vi "Global Variables.vi"() -> ()   [LabVIEW 2012]
panel:
  in  "Pivots Enabled?":bool=TRUE
  in  "Climbing":bool
  in  "Caterpillar Back":bool
  in  "Caterpillar ON":bool
  in  "J2 Xbox RB":bool
  in  "J2 Xbox B":bool
  in  "J2 Xbox Y":bool
  in  "J1 Xbox B":bool
  in  "J2 Xbox X":bool
  in  "J1 Xbox Y":bool
  in  "Climb Shoot Motor":dbl
  in  "J1 Xbox X":bool
  in  "J2 Xbox LB":bool
  in  "J2 Xbox A":bool
  in  "J2 Xbox Select":bool
  in  "J1 Xbox Select":bool
  in  "J1 Xbox LB":bool
  in  "J1 Xbox RB":bool
  in  "J1 Xbox A":bool
  in  "ICE BR":dbl
  in  "ICE BL":dbl
  in  "ICE FR":dbl
  in  "ICE FL":dbl
  in  "Konami":bool
  in  "Calibration BR":dbl
  in  "Calibration BL":dbl
  in  "Calibration FR":dbl
  in  "Calibration FL":dbl
  in  "Rotational Motor BR":dbl
  in  "Rotational Motor BL":dbl
  in  "Rotational Motor FR":dbl
  in  "Rotational Motor FL":dbl
  in  "Drive Motor BR":dbl
  in  "Drive Motor BL":dbl
  in  "Drive Motor FR":dbl
  in  "Drive Motor FL":dbl
  # "Steering"
  # "Drive"
  # "Calibration"
  # "ICE Calibrate"
  # "Buttons"
  # "ICE"
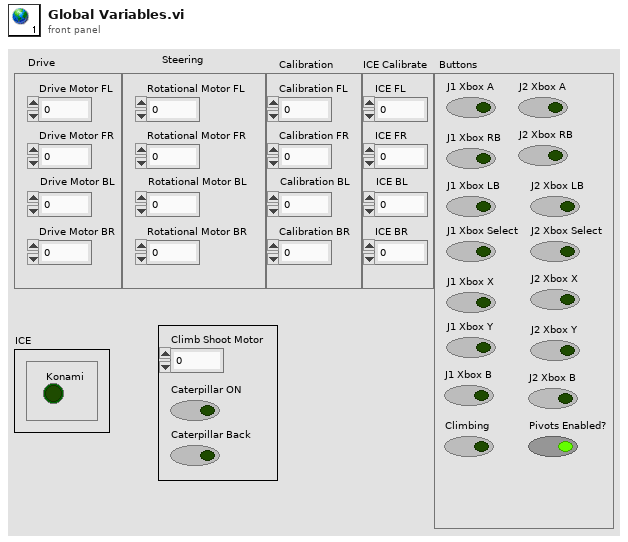
[diagram p1: front panel]
diagram:
